vi "SingleCounter.vi"(8 "error in":errorcluster, 11 "Dwell_time_ms":dbl=100.0 format="%.3f") -> (0 "error out":errorcluster, 2 "counts/s":dbl=10.0, 3 "counts":u32=1)   [LabVIEW 2018]
doc: "I. Description:\nThis example demonstrates how to count digital events on a Counter Input Channel. The Initial Count, Count Direction, and Edge are all configurable. This example also shows how to use a secondary counter and a digital input line to count events for a specified amount of time, following an external digital trigger.\n\nEdges are counted on the primary counter's default input terminal (refer to section IV, I/O Connections Overview, for more information), but it could easily be modified to count edges on a PFI or RTSI line. \n\nII. Instructions for Running:\n1. Select the Physical Channel that corresponds to the counter you want to count edges on the DAQ device. (This counter is called the Input Counter.)\n2. Enter the Initial Count, Count Direction, and measurement Edge to specify how you want the counter to count. Additionally, you can change the input terminal where events are counted using the channel property node.\n3. Select the Physical Channel that corresponds to the secondary counter you want to generate a single pulse on the DAQ device. (This counter is called the Gating Counter.)\n4. Enter the Gate Length, Idle State, and Initial Delay to specify how you want the gate signal to be generated.\n5. Select the source for the Digital Start Trigger and the on which to trigger.\n\nIII. Block Diagram Steps:\n1. Create a Counter Input channel to Count Events. The Edge parameter is used to determine if the counter will increment on rising or falling edges.\n2. Create a Counter Output channel to produce a Pulse in terms of Time. If the Idle State of the pulse is set to low, the state of the line will begin low and remain low after the generation is stopped.\n3. Call the DAQmx Start Trigger VI to configure the pulse to begin on a digital trigger.\n4. Call the Start VI in each task to arm the counters and begin counting or generating. The input counter will be preloaded with the Initial Count. The pulse will not begin until the generating counter receives a digital trigger and after the Initial Delay (in seconds) has expired.\n5. Use the Wait Until Done VI to ensure the entire gate pulse is generated before ending the task.\n6. Call the DAQmx Read VI to poll the input counter after the gate pulse generation has finished.\n7. Call the Clear Task VI to clear each Task.\n8. Use the popup dialog box to display an error, if any.\n\nIV. I/O Connections Overview:\nThe input counter will count edges on the input terminal of the counter specified in the left Physical Channel I/O control. The gating counter will generate a digital pulse on the output terminal of the counter specified in the right Physical Channel I/O control. Connect the default output line of the gating counter to the default gate line of the input counter. This will allow the gating counter to control when the input counter can count events.\n\nIn this example the input counter will count edges on the default input terminal on ctr0, and the gating counter will generate a digital pulse on the default output terminal on ctr1. Connect your start trigger source to the appropriate connection specified by \"Start Trigger Source\" on the front panel. \n\nFor more information on the default counter input and output terminals for your device, open the NI-DAQmx Help, and refer to Counter Signal Connections found under the Device Considerations book in the table of contents."
uses:
  <vilib>/DAQmx/read.llb/DAQmx Read (Counter U32 1Chan 1Samp).vi
  GLOBAL_VAR.vi
  <vilib>/DAQmx/create/channels.llb/DAQmx Create Channel (CI-Count Edges).vi
  <vilib>/DAQmx/create/channels.llb/DAQmx Create Channel (CO-Pulse Generation-Time).vi
  <vilib>/DAQmx/configure/timing.llb/DAQmx Timing (Implicit).vi
  <vilib>/DAQmx/miscellaneous.llb/DAQmx Fill In Error Info.vi
  <resource>/objmgr/daqmx.rc
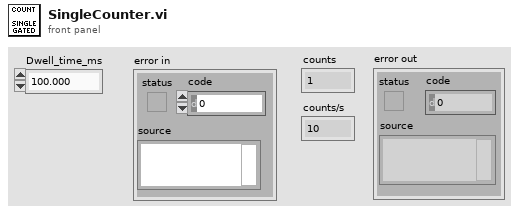
[diagram p1: front panel]
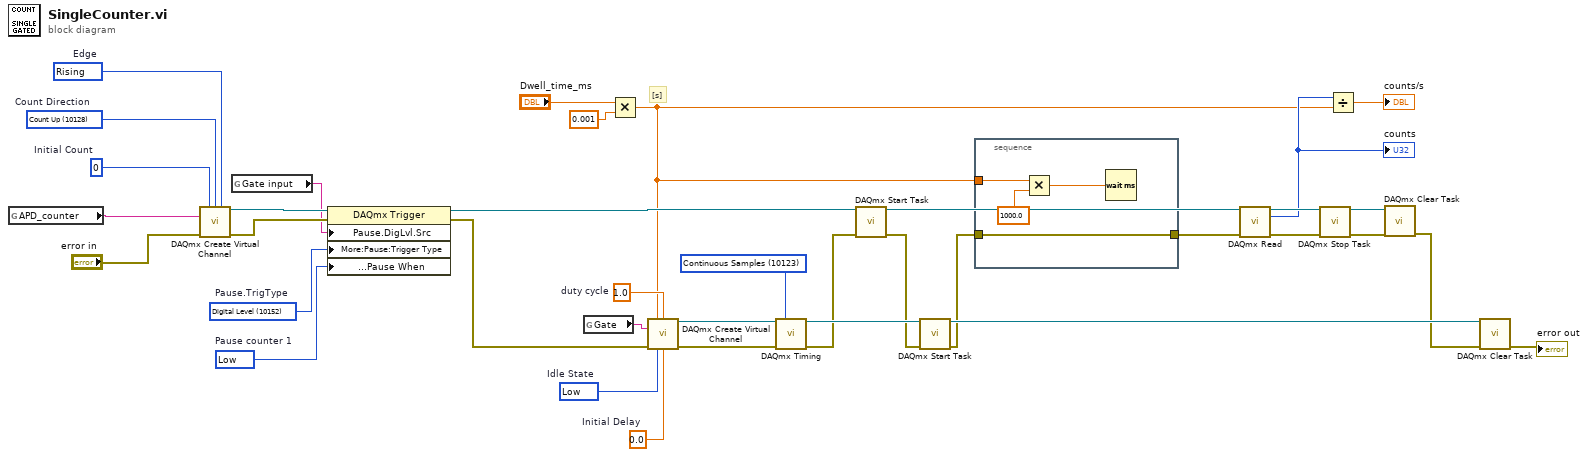
[diagram p0: block diagram]
diagram:
  w26 = 10214 items=["High"=10192, "Low"=10214]  # Pause counter 1
  w28 = 1.0  # duty cycle
  w29 = 10123 items=["Finite Samples"=10178, "Continuous Samples"=10123, "Hardware Timed Single Point"=12522] ("sample mode")
  w33 = 0.0  # Initial Delay
  w34 = 10214 items=["High"=10192, "Low"=10214]  # Idle State
  w35 = u32 0  # Initial Count
  w36 = 10128 items=["Count Up"=10128, "Count Down"=10124, "Externally Controlled"=10326]  # Count Direction
  w37 = 10280 items=["Rising"=10280, "Falling"=10171]  # Edge
  w7 = 10152 items=["Analog Level"=10101, "Analog Window"=10103, "Digital Level"=10152, "Digital Pattern"=10398, "None"=10230]  # Pause.TrigType
  # "[s]"
  n1 = global read "GLOBAL_VAR.vi" "APD_counter"() -> (w6:tag)
  n2 = call-poly <vilib>:"DAQmx Create Virtual Channel.vi"("initial count"=w35, "count direction"=w36, "edge"=w37, "counter"=w6, "error in"="error in") -> ("task out"=w24:refnum<k21>, "error out"=w25:errorcluster)  [unwired: 9 in]
  n3 = global read "GLOBAL_VAR.vi" "Gate input"() -> (w5:tag)
  n4 = property class="DAQmx Trigger"(reference=w24, error in=w25, "Pause.DigLvl.Src"=w5, "More:Pause:Trigger Type"=w7, "More:Pause:Digital Level:Pause When"=w26) -> (reference out=w27:refnum<k21>, error out=w17:errorcluster)
  n5 = global read "GLOBAL_VAR.vi" "Gate"() -> (w4:tag)
  n6 = Multiply(x="Dwell_time_ms", y=0.001) -> (x*y=w2:dbl)
  n7 = call-poly <vilib>:"DAQmx Create Virtual Channel.vi"("high time"=w2, "low time"=w28, "counter"=w4, "error in"=w17, "idle state"=w34, "initial delay"=w33) -> ("task out"=w30:refnum<k21>, "error out"=w32:errorcluster)  [unwired: 8 in]
  n8 = call-poly <vilib>:"DAQmx Timing.vi"("task/channels in"=w30, "sample mode"=w29, "error in"=w32) -> ("task out"=w31:refnum<k21>, "error out"=w13:errorcluster)  [unwired: 11 in]
  n9 = call <vilib>:"DAQmx Start Task.vi"("task/channels in"=w27, "error in"=w13) -> ("task out"=w21:refnum<k21>, "error out"=w12:errorcluster)  [unwired: 12 in]
  n10 = call <vilib>:"DAQmx Start Task.vi"("task/channels in"=w31, "error in"=w12) -> ("task out"=w23:refnum<k21>, "error out"=w11:errorcluster)  [unwired: 12 in]
  n11 = stacked-sequence {
    tunnel: [w41] -> w20
    tunnel: w11 -> [w41]
    tunnel: w2 -> [w38]
    frame #0 {
      n12 = Multiply(x=w38, y=1000.0) -> (x*y=w40:dbl)
      n13 = Wait (ms)(milliseconds to wait=w40) -> ()  [unwired: 1 out]
    }
  }
  n14 = call-poly <vilib>:"DAQmx Read.vi"("task/channels in"=w21, "error in"=w20) -> ("task out"=w19:refnum<k21>, "data"=w18:u32, "error out"=w16:errorcluster)  [unwired: 11 in]
  "counts" <- w18
  n15 = call <vilib>:"DAQmx Stop Task.vi"("task/channels in"=w19, "error in"=w16) -> ("task out"=w22:refnum<k21>, "error out"=w15:errorcluster)  [unwired: 12 in]
  n16 = Divide(x=w18, y=w2) -> (x/y=→"counts/s":dbl)
  n17 = call <vilib>:"DAQmx Clear Task.vi"("task in"=w22, "error in"=w15) -> ("error out"=w14:errorcluster)  [unwired: 13 in]
  n18 = call <vilib>:"DAQmx Clear Task.vi"("task in"=w23, "error in"=w14) -> ("error out"=→"error out":errorcluster)  [unwired: 13 in]
